vi "wrap.vi"(1 "Degrees In":dbl) -> (0 "Degrees Out":dbl)   [LabVIEW 2018]
doc: "This VI Wraps phase data to stay between 180 and -180 degrees."
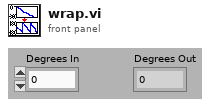
[diagram p1: front panel]
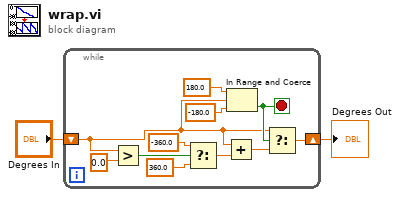
[diagram p0: block diagram]
diagram:
  n1 = while {
    shift-right: [w3] -> w2
    shift-left: "Degrees In" -> [w5]
    stop <- w6 stop-if-true
    n2 = Greater?(x=w5, y=0.0) -> (0:w12:bool)
    n3 = Select(t=-360.0, s=w12, f=360.0) -> (s? t:f=w9:dbl)
    n4 = Add(x=w5, y=w9) -> (x+y=w4:dbl)
    n5 = In Range and Coerce(upper limit=180.0, x=w5, lower limit=-180.0) -> (In Range?=w6:bool)  [unwired: 1 out]
    n6 = Select(t=w5, s=w6, f=w4) -> (s? t:f=w3:dbl)
  }
  "Degrees Out" <- w2
